vi "kf_demod_update.vi"(4 "Unlocked":bool, 6 "Reset":bool, 8 "Variance":dbl[](array[numeric]), 9 "KF in":T1 {"K" format="%#_3g"; "y lim" format="%#_3g"; "x lim" format="%#_3g"; "P" format="%#_3g"; "H" format="%#_3g"; "x" format="%#_3g"; "Q" format="%#_3g"; "R" format="%#_3g"; "B" format="%#_3g"; "A" format="%#_3g"}, 10 "Config":T3={"IO params"={"Conversion"={"Rate"=4.0, "In channels"=2, "Out channels"=4}, "Carriers"={"Phase shift"=180.0, "Levels"=[[0.8, 0.8, 0.8], [0.03, 0.03, 0.03]], "Delay samples"=73.15}}, "High rate STFT"={"Win param"=101.5, "Window type"=61, "Win order"=2, "DFT size"=64, "Channels"=[7], "Oversample"=64}, "Low rate STFT"={"Win param"=120.0, "Window type"=61, "Win order"=8, "DFT size"=64, "Channels"=[7], "Oversample"=64}, "Filtering"={"Hum"={"Frequency"=0.0, "Tc"=0.0, "Limit"=101.5, "FFT filter"=FALSE, "Detrend mode"=enum."Robust linear", "Enable"=FALSE}, "Kalman"={"Process noise"=101.5, "Measure noise"=101.5, "Unlock m noise"=101.5, "Mode"=enum."FFT"}, "Distortion"={"LF cut"=101.5, "Tc"=3.0, "Limit"=101.5, "FFT filter"=FALSE, "Detrend mode"=enum."Robust linear", "Enable"=FALSE}, "Lowpass"={"Frequency"=0.0, "Order"=0, "Enable"=FALSE}, "Impulse"={"Win order"=102, "Locked limit"=101.5, "Locked count"=102, "Threshold Tc"=101.5, "Thresh sigmas"=101.5, "Thresh min"=101.5, "After"=0, "Detrend"=FALSE, "Enable"=FALSE}}} {"Filtering"."Impulse"."Thresh min" format="%#_3p"; "Filtering"."Impulse"."Threshold Tc" format="%#_3p"; "Filtering"."Impulse"."Locked limit" format="%#_3p"; "Filtering"."Impulse"."Thresh sigmas" format="%#_3p"; "Filtering"."Lowpass"."Frequency" format="%#_4p"; "Filtering"."Distortion"."Limit" format="%#_3p"; "Filtering"."Distortion"."LF cut" format="%#_3p"; "Filtering"."Kalman"."Unlock m noise" format="%#_3p"; "Filtering"."Kalman"."Measure noise" format="%#_3p"; "Filtering"."Kalman"."Process noise" format="%#_3p"; "Filtering"."Hum"."Limit" format="%#_3p"; "Filtering"."Hum"."Frequency" format="%#_4p"; "Low rate STFT"."Oversample" min=1 step=1; "Low rate STFT"."Channels" min=0 step=1; "Low rate STFT"."DFT size" min=1 step=1; "Low rate STFT"."Window type" items=["Rectangle"=0, "Hanning"=1, "Hamming"=2, "Blackman-Harris"=3, "Exact Blackman"=4, "Blackman"=5, "Flat Top"=6, "4 Term B-Harris "=7, "7 Term B-Harris"=8, "Low Sidelobe"=9, "Blackman Nuttall"=11, "Triangle"=30, "Bartlett-Hanning"=31, "Bohman"=32, "Parzen"=33, "Welch"=34, "Kaiser"=60, "Dolph-Chebyshev"=61, "Gaussian"=62]; "High rate STFT"."Oversample" min=1 step=1; "High rate STFT"."Channels" min=0 step=1; "High rate STFT"."DFT size" min=1 step=1; "High rate STFT"."Window type" items=["Rectangle"=0, "Hanning"=1, "Hamming"=2, "Blackman-Harris"=3, "Exact Blackman"=4, "Blackman"=5, "Flat Top"=6, "4 Term B-Harris "=7, "7 Term B-Harris"=8, "Low Sidelobe"=9, "Blackman Nuttall"=11, "Triangle"=30, "Bartlett-Hanning"=31, "Bohman"=32, "Parzen"=33, "Welch"=34, "Kaiser"=60, "Dolph-Chebyshev"=61, "Gaussian"=62]; "IO params"."Carriers"."Levels" min=0.0 step=0.1; "IO params"."Conversion"."Rate" format="%#_8g"}, 11 "Error":dbl[](array[numeric])) -> (1 "KF out":T1 {"K" format="%#_3g"; "y lim" format="%#_3g"; "x lim" format="%#_3g"; "P" format="%#_3g"; "H" format="%#_3g"; "x" format="%#_3g"; "Q" format="%#_3g"; "R" format="%#_3g"; "B" format="%#_3g"; "A" format="%#_3g"}, 3 "New amplitudes":cdb[](array[numeric]) format="%_3p")   [LabVIEW 2014]
uses:
  ilemt_config.ctl
  IO_params.ctl
  stft_params.ctl
  <vilib>/Analysis/4window.llb/windowTd.ctl
  filter_params.ctl
  detrend_mode.ctl
  utilities/kalman_filter.ctl
  <vilib>/Analysis/Matrix/Datatypes/RealMatrix.ctl
  <vilib>/Analysis/Matrix/Numeric/Conversions/Array To Matrix - RA2.vi
  <vilib>/Analysis/Matrix/NI_Matrix.lvlib
  <vilib>/Analysis/NI_AALPro.lvlib
panel:
  out "Measurement amplitudes":cdb[](array[numeric]) format="%_3p"
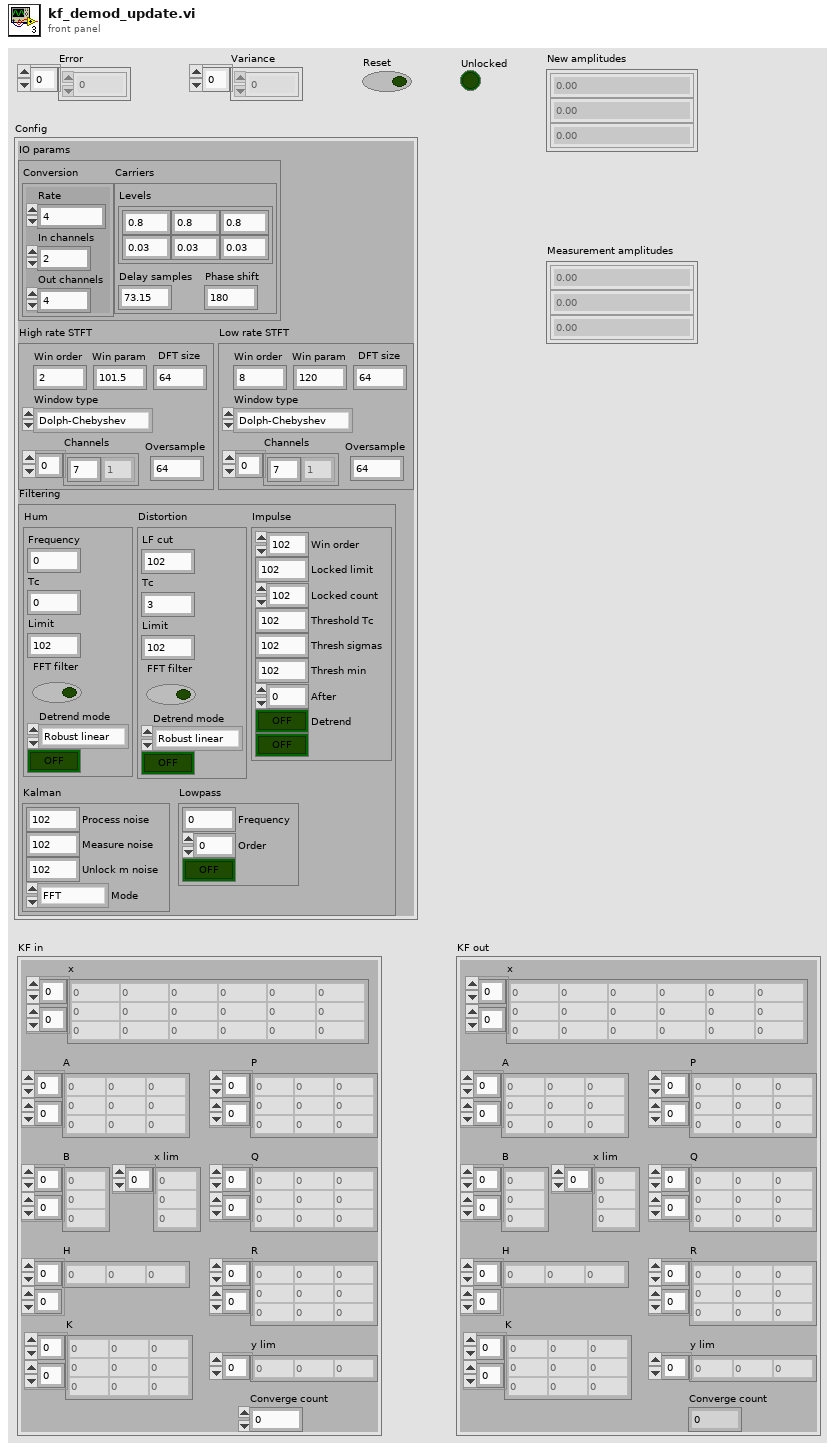
[diagram p1: front panel]
types:
  T1 = typedef "kalman_filter.ctl" = cluster{"A":T2, "B":T2, "H":T2, "Q":T2, "R":T2, "x":T2, "P":T2, "x lim":dbl[], "y lim":dbl[], "K":T2, "Converge count":i32}
  T2 = typedef "NI_Matrix.lvlib/RealMatrix.ctl" = dbl[][]
  T3 = typedef "ilemt_config.ctl" = cluster{"IO params":T4, "High rate STFT":T5, "Low rate STFT":T5, "Filtering":T7}
  T4 = typedef "IO_params.ctl" = cluster{"Conversion":cluster{"Rate":dbl, "In channels":u32, "Out channels":u32}, "Carriers":cluster{"Phase shift":dbl, "Levels":dbl[][], "Delay samples":dbl}}
  T5 = typedef "stft_params.ctl" = cluster{"Win param":dbl, "Window type":T6, "Win order":i32, "DFT size":i32, "Channels":i32[], "Oversample":i32}
  T6 = typedef "NI_AALPro.lvlib/windowTd.ctl" = u32
  T7 = typedef "filter_params.ctl" = cluster{"Hum":cluster{"Frequency":dbl, "Tc":dbl, "Limit":dbl, "FFT filter":bool, "Detrend mode":T8, "Enable":bool}, "Kalman":cluster{"Process noise":dbl, "Measure noise":dbl, "Unlock m noise":dbl, "Mode":enum16{"FFT", "KF demod"}}, "Distortion":cluster{"LF cut":dbl, "Tc":dbl, "Limit":dbl, "FFT filter":bool, "Detrend mode":T8, "Enable":bool}, "Lowpass":cluster{"Frequency":dbl, "Order":i32, "Enable":bool}, "Impulse":cluster{"Win order":i32, "Locked limit":dbl, "Locked count":i32, "Threshold Tc":dbl, "Thresh sigmas":dbl, "Thresh min":dbl, "After":i32, "Detrend":bool, "Enable":bool}}
  T8 = typedef "detrend_mode.ctl" = enum16{"Zero mean", "Linear", "Robust linear"}
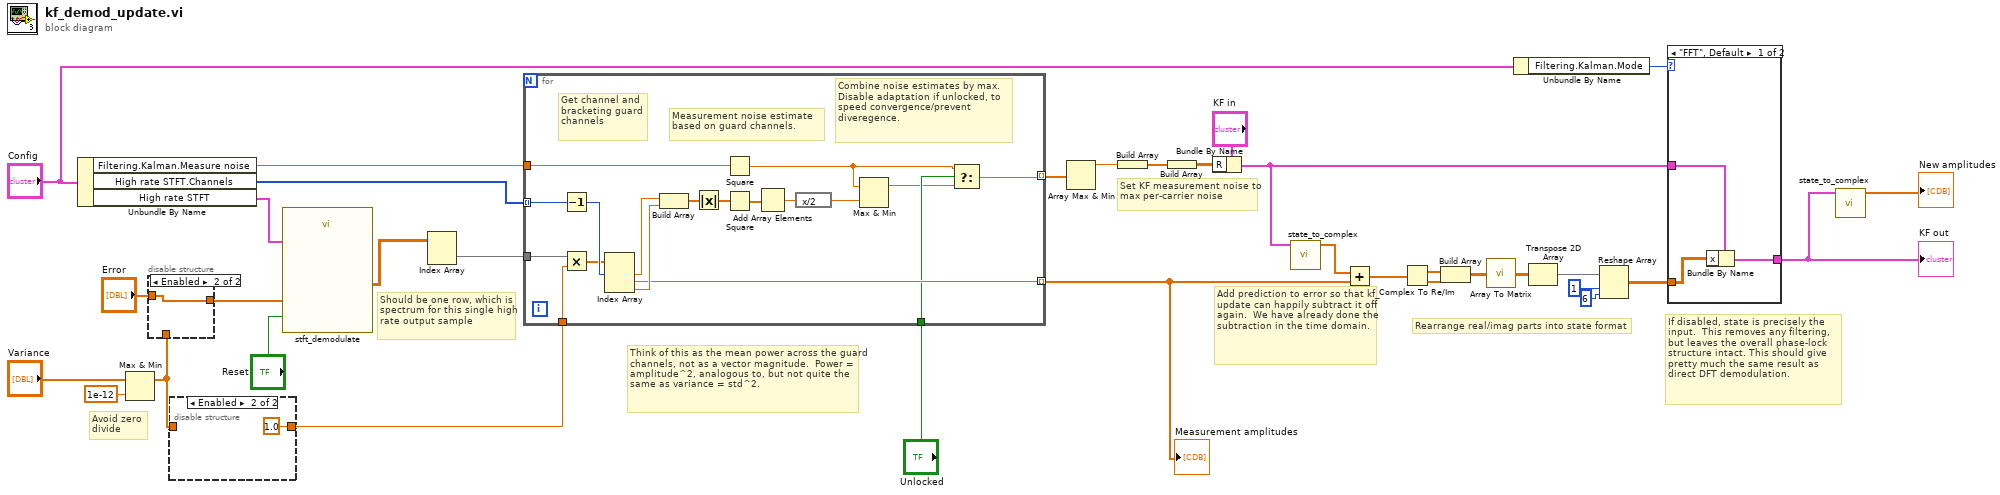
[diagram p0: block diagram]
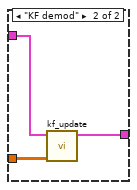
[diagram p2: hidden frame]
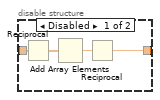
[diagram p3: hidden frame]
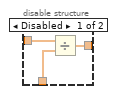
[diagram p4: hidden frame]
diagram:
  # "Think of this as the mean power across the guard channels, not as a vector magnitude.  Power = amplitude^2, analogous to, but not quite the same as variance = std^2."
  # "Rearrange real/imag parts into state format"
  # "Set KF measurement noise to max per-carrier noise"
  # "If disabled, state is precisely the input.  This removes any filtering, but leaves the overall phase-lock structure intact. This should give pretty much the same result as direct DFT demodulation."
  # "Avoid zero divide"
  # "Add prediction to error so that kf_update can happily subtract it off again.  We have already done the subtraction in the time domain."
  # "Should be one row, which is spectrum for this single high rate output sample"
  n1 = Unbundle By Name("Config") -> ("Filtering.Kalman.Measure noise"=w17:dbl, "High rate STFT.Channels"=w12:i32[], "High rate STFT"=w18:T5)
  n2 = Max & Min(x="Variance", y=1e-12 ("sum")) -> (max(x,y)=w20:dbl[])  [unwired: 1 out]
  n3 = disable-structure shown="Enabled" {
    disable-tunnel: "Error" -> [w37 w38]
    disable-tunnel: [w36 w38] -> w31
    disable-tunnel: w20 -> [w35 _]
    frame Disabled {
      n4 = Divide(x=w37, y=w35) -> (x/y=w36:dbl[])
    }
    frame Enabled {
    }
  }
  n5 = disable-structure shown="Enabled" {
    disable-tunnel: w20 -> [w41 _]
    disable-tunnel: [w39 1.0] -> w19
    frame Disabled {
      n6 = Reciprocal(x=w41) -> (1/x=w42:dbl[])
      n7 = Add Array Elements(numeric array=w42) -> (sum=w40:dbl)
      n8 = Reciprocal(x=w40) -> (1/x=w39:dbl)
    }
    frame Enabled {
    }
  }
  n9 = call "stft_demodulate.vi"("STFT params"=w18, "Reset"="Reset", "X"=w31) -> ("STFT"=w11:cdb[][])  [unwired: 6 in, 2 out]
  n10 = Index Array(array=w11) -> (element=w10:cdb[])  [unwired: 2 in]
  n11 = for {
    tunnel: w19 -> [w55]
    tunnel: [w50] -> w7 mode=indexing
    tunnel: "Unlocked" -> [w48]
    tunnel: w10 -> [w45]
    tunnel: w12 -> [w44] mode=indexing
    tunnel: w17 -> [w53]
    tunnel: [w46] -> w9 mode=indexing
    # "Combine noise estimates by max.  Disable adaptation if unlocked, to speed convergence/prevent diveregence."
    # "Measurement noise estimate based on guard channels."
    # "Get channel and bracketing guard channels"
    n12 = Decrement(x=w44) -> (x-1=w61:i32)
    n13 = Multiply(x=w45, y=w55) -> (x*y=w56:cdb[])
    n14 = Index Array(array=w56, index #1=w61) -> (element #1=w60:cdb, element #2=w50:cdb, element #3=w59:cdb)  [unwired: 2 in]
    n15 = Build Array(w60, w59) -> (w52:cdb[])
    n16 = Absolute Value(x=w52) -> (abs(x)=w51:dbl[])
    n17 = Square(x=w53) -> (x^2=w49:dbl)
    n18 = Square(x=w51) -> (x^2=w57:dbl[])
    n19 = Add Array Elements(numeric array=w57) -> (sum=w58:dbl)
    n20 = expression code="x/2"(w58) -> (w54:dbl)
    n21 = Max & Min(x=w49, y=w54) -> (max(x,y)=w47:dbl)  [unwired: 1 out]
    n22 = Select(t=w49, s=w48, f=w47) -> (s? t:f=w46:dbl)
  }
  "Measurement amplitudes" <- w7
  n23 = Array Max & Min(array=w9) -> (max value=w8:dbl)  [unwired: 3 out]
  n24 = Build Array(w8) -> (w24:dbl[])
  n25 = Build Array(w24) -> (w23:T2)
  n26 = Bundle By Name(cluster="KF in", "R"=w23) -> (w14:T1)
  n27 = call "state_to_complex.vi"("KF in"=w14) -> ("Amplitudes"=w27:cdb[])  [unwired: 10 in]
  n28 = Add(x=w27, y=w7) -> (x+y=w26:cdb[])
  n29 = Complex To Re/Im(x + iy=w26) -> (x=w29:dbl[], y=w28:dbl[])
  n30 = Build Array(w29, w28) -> (w5:dbl[][])
  n31 = call-poly <vilib>:"Array To Matrix.vi"("Real 2D Array"=w5) -> ("Real Matrix"=w4:T2)
  n32 = Unbundle By Name("Config") -> ("Filtering.Kalman.Mode"=w15:enum16{"FFT", "KF demod"})
  n33 = Transpose 2D Array(2D array=w4) -> (transposed array=w6:T2)
  n34 = Reshape Array(w6, 1 ("dimension size"), 6 ("dimension size")) -> (w1:T2)
  n35 = case shown="\"FFT\", Default" w15 {
    tunnel: [w63 w67] -> w34
    tunnel: w1 -> [w64 w66]
    tunnel: w14 -> [w62 w65]
    frame "FFT", Default {
      n36 = Bundle By Name(cluster=w62, "x"=w64) -> (w63:T1)
    }
    frame "KF demod" {
      n37 = call "kf_update.vi"("z"=w66, "KF in"=w65) -> ("KF out"=w67:T1)  [unwired: 8 in, 1 out]
    }
  }
  "KF out" <- w34
  n38 = call "state_to_complex.vi"("KF in"=w34) -> ("Amplitudes"=→"New amplitudes":cdb[])  [unwired: 10 in]
